vi "vPage_9205x1_CHx4.vi"() -> ()   [LabVIEW 2022 SP3]
uses:
  <vilib>/Utility/sysdir.llb/System Directory Type.ctl
  <vilib>/express/express analysis/Spectral/Block/exnSpectralBlock spectral measurements peak poly.vi
  <vilib>/express/express analysis/Spectral/Block/exnSpectralBlock spectral measurements peak DDT.vi
  <vilib>/express/express analysis/Spectral/XNode/ExpressSpectralMeasurementsBlockNode.xnode
panel:
  in  "Show_FFT":bool
  in  "Show":bool
  in  "¸ê®Æ§¨\nµù°O>":string
  in  "Filter(Hz)\nLow-Cut":dbl=10.0
  out "DAQ Stoped":bool
  in  "SW \n(C1)":bool[](array[boolean])=[TRUE, TRUE, TRUE, TRUE, TRUE, TRUE, TRUE, TRUE]
  in  "Sample \nto Read":i32=6400
  in  "Sample\nRate":dbl=6400.0
  in  "Enable Saving":bool
  in  "Stop":bool
  out "C1-Save":bool
  out "C1-Trigger":bool
  out "C1":i32
  out "C1-All":dynamicdata(graph)
  out "C1-0":dynamicdata(graph)
  out "C1-2":dynamicdata(graph)
  out "C1-1":dynamicdata(graph)
  out "C1-3":dynamicdata(graph)
  # "使用前請先確認 \nDAQ 擷取卡設定"
  # "本頁畫面顯示為 觸發後訊號"
  # "FFT Filter by useing High-pass with Lower Cut-Off (Hz)"
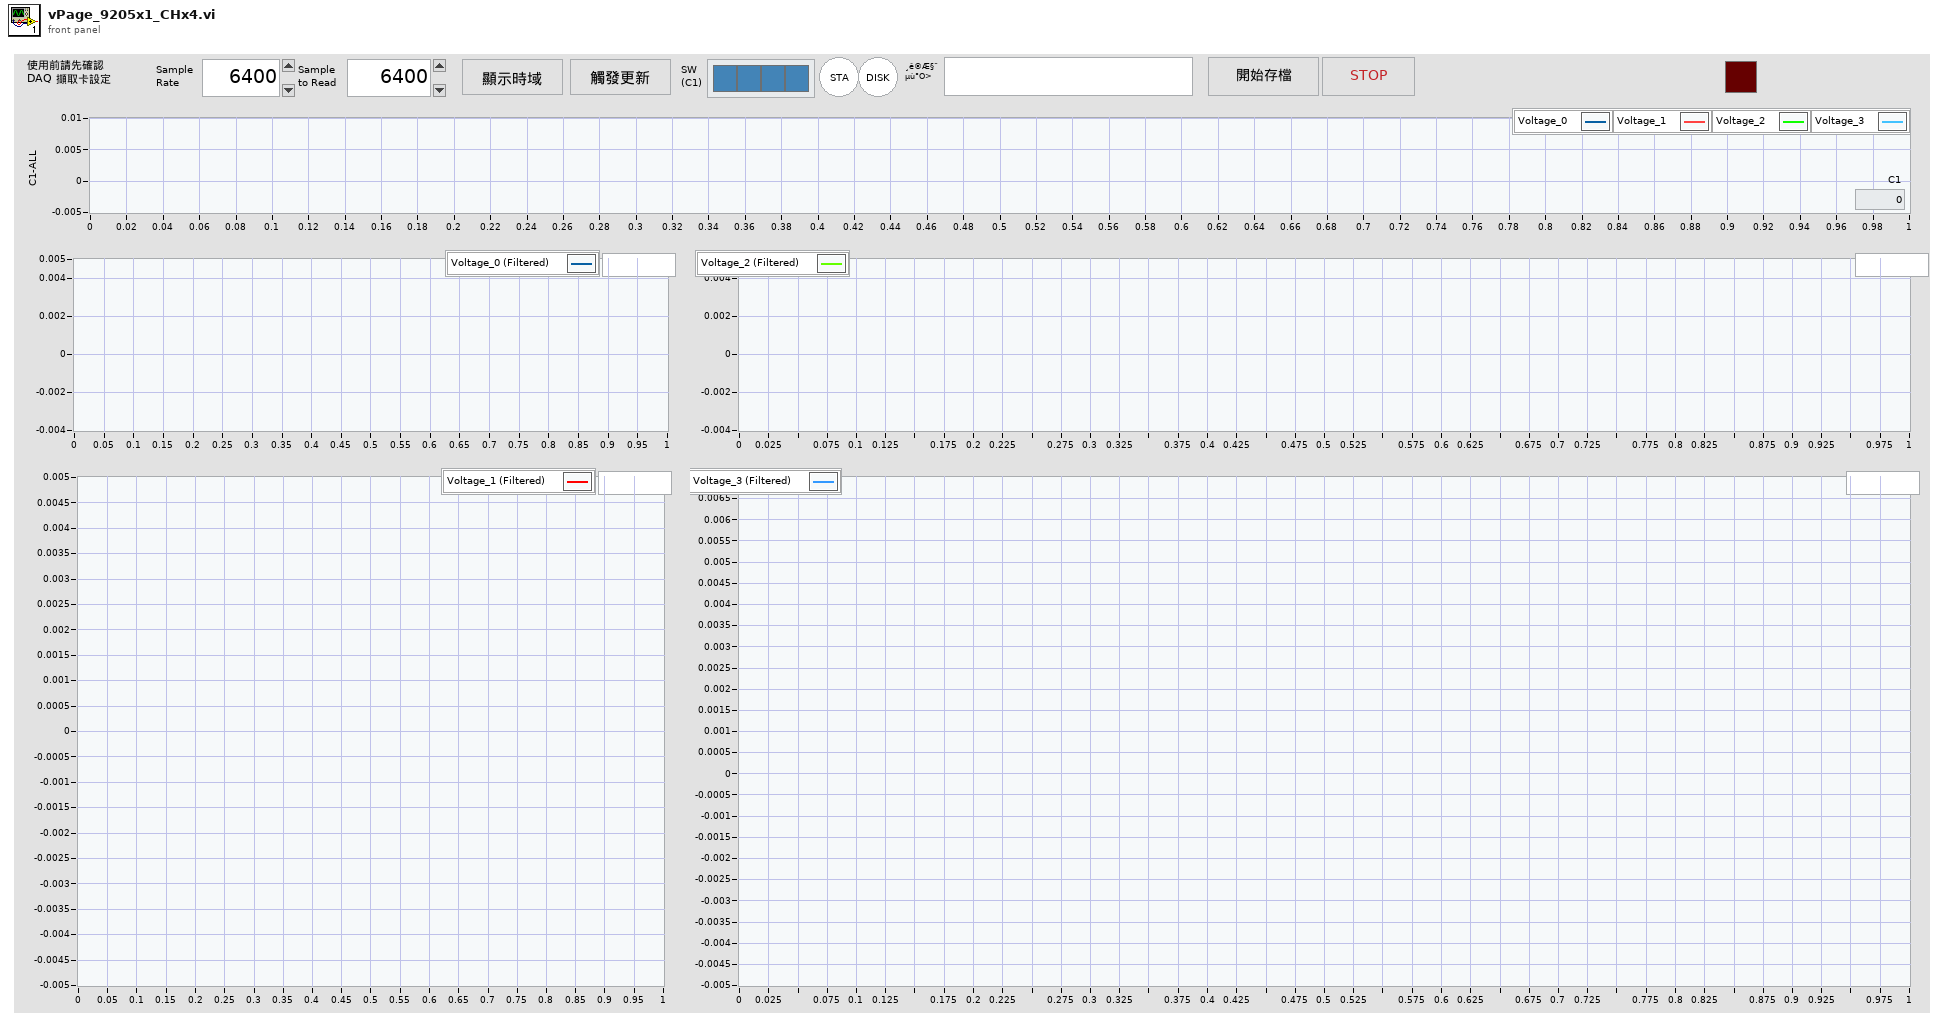
[diagram p1: front panel]
types:
  T1 = enum8{"Enabled", "Disabled", "Disabled and Grayed Out"}
  T2 = typedef "System Directory Type.ctl" = i32
  T3 = cluster{"task out":refnum<k21>, "data":dynamicdata}
  T4 = cluster{"averaging mode":u16, "weighting mode":u16, "number of averages":u32}
  T5 = cluster{"dB On (F)":bool, "unwrap phase (F)":bool, "convert to degree (F)":bool}
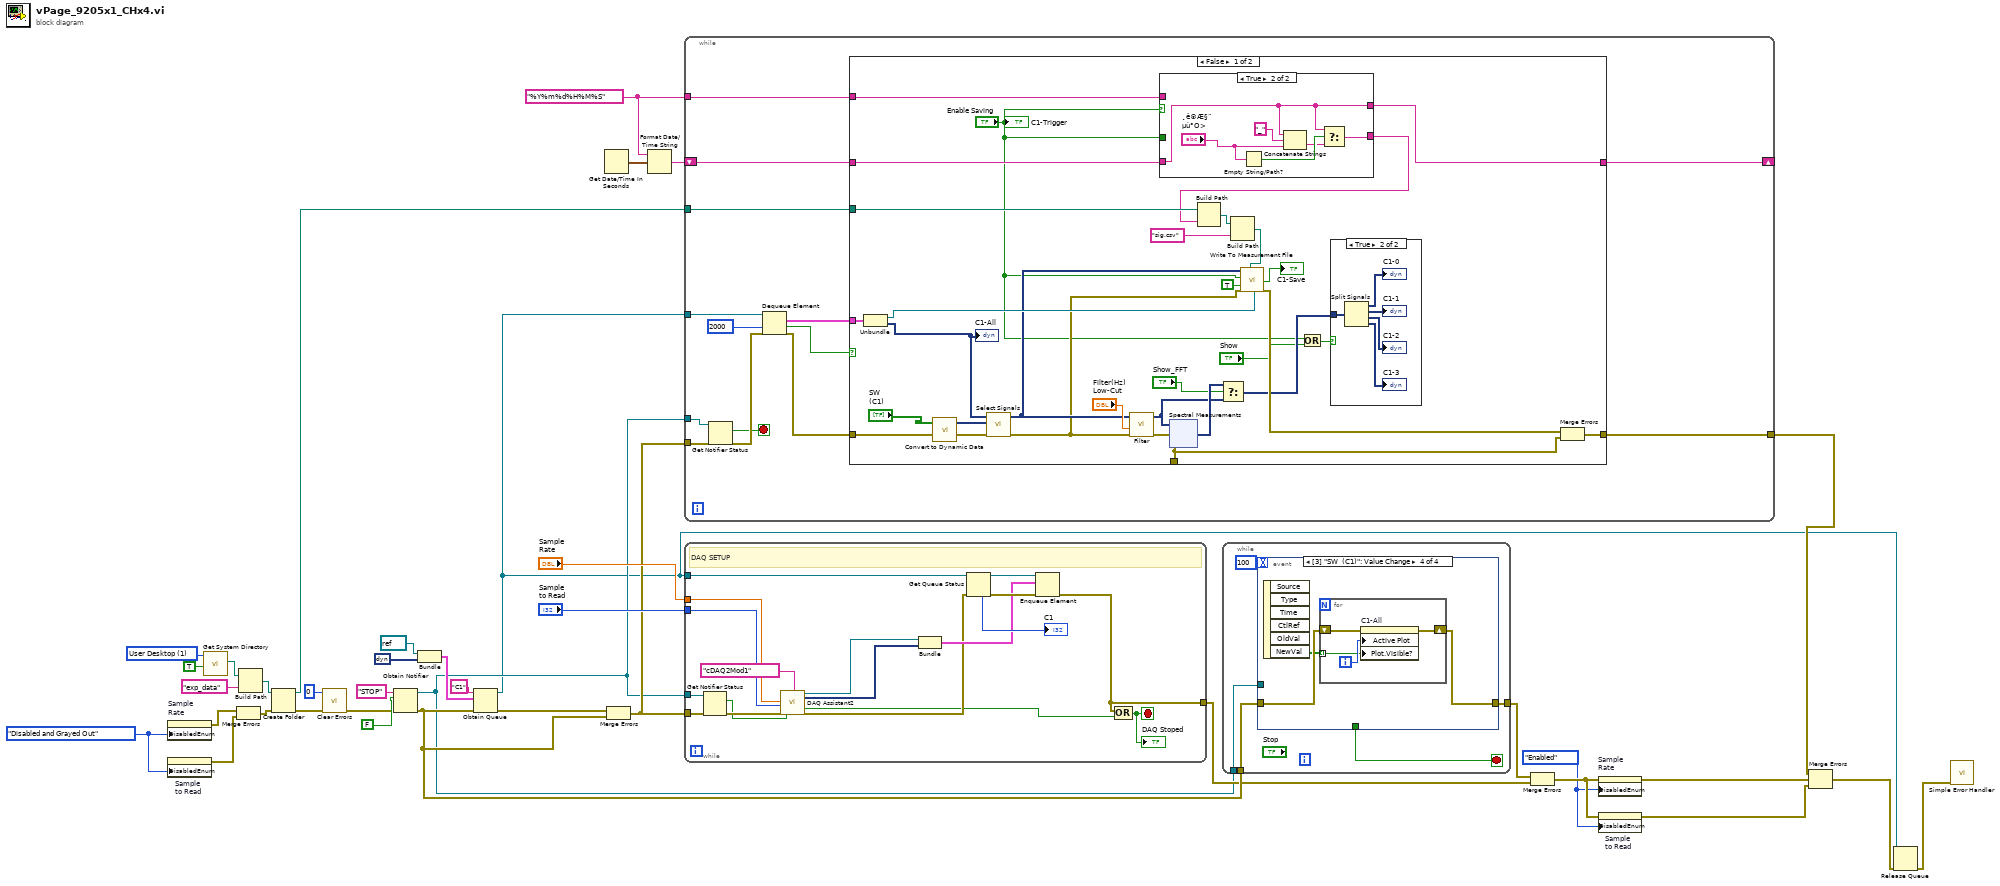
[diagram p0: block diagram]
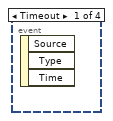
[diagram p2: hidden frame]
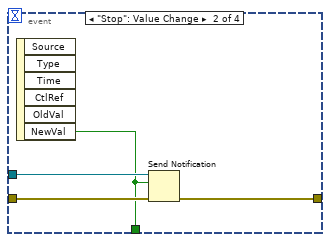
[diagram p3: hidden frame]
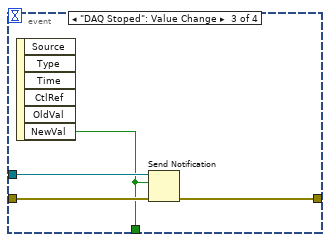
[diagram p4: hidden frame]
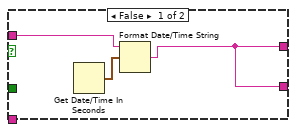
[diagram p6: hidden frame]
diagram:
  w7 = T1."Enabled" ("Disabled")
  w12 = T1."Disabled and Grayed Out" ("Disabled")
  w13 = "%Y%m%d%H%M%S" ("time format string (%c)")
  w23 = T2 1 items=["User Home"=0, "User Desktop"=1, "User Documents"=2, "User Application Data"=3, "User Preferences"=4, "User Temporary"=5, "Public Documents"=6, "Public Application Data"=7, "Public Preferences"=8, "Public Cache"=13, "System Core Libraries"=9, "System Installed Libraries"=10, "Application Files"=11, "Boot Volume Root"=12] ("system directory type")
  n1 = property on="Sample\nRate" class="DigNum (strict)"("DisabledEnum"=w12) -> (error out=w11:errorcluster)  [unwired: 2 in, 1 out]
  n2 = property on="Sample \nto Read" class="DigNum (strict)"("DisabledEnum"=w12) -> (error out=w9:errorcluster)  [unwired: 2 in, 1 out]
  n3 = call <vilib>:"Get System Directory.vi"("create directory if not found? (F)"=TRUE, "system directory type"=w23) -> ("system directory"=w25:path)  [unwired: 9 in]
  n4 = Merge Errors(w11, w9) -> (w10:errorcluster)
  n5 = Build Path(base path=w25, name or relative path="exp_data") -> (appended path=w19:path)
  n6 = Create Folder(path (use dialog)=w19, error in=w10) -> (created path=w18:path, error out=w21:errorcluster)  [unwired: 1 in, 1 out]
  n7 = call <vilib>:"Clear Errors.vi"("error in (no error)"=w21, "specific error code to clear (0: all)"=0) -> ("error out"=w20:errorcluster)  [unwired: 4 in, 1 out]
  n8 = Obtain Notifier(name (unnamed)="STOP", notification data type=FALSE, error in (no error)=w20) -> (notifier out=w14:refnum<notifier>, error out=w17:errorcluster)  [unwired: 1 in, 1 out]
  n9 = Bundle("task out"=refnum<k21> refnum, "data"=dynamicdata []) -> (w30:T3)  [unwired: 1 in]
  n10 = Obtain Queue(name (unnamed)="C1", element data type=w30, error in (no error)=w17) -> (queue out=w1:refnum<queue>, error out=w38:errorcluster)  [unwired: 2 in, 1 out]
  n11 = Get Date/Time In Seconds() -> (seconds since 1Jan1904=w28:timestamp)
  n12 = Merge Errors(w38, w17) -> (w29:errorcluster)
  n13 = Format Date/Time String(time format string (%c)=w13, seconds (now)=w28) -> (date/time string=w27:string)  [unwired: 1 in]
  n14 = while {
    tunnel: w29 -> [w52]
    tunnel: w14 -> [w50]
    tunnel: w1 -> [w49]
    shift-right: [w39] -> _
    shift-left: w27 -> [w43]
    tunnel: w18 -> [w44]
    tunnel: [w40] -> w2
    tunnel: w13 -> [w42]
    stop <- w47 stop-if-true
    n15 = Get Notifier Status(notifier=w50, error in (no error)=w52) -> (current notification=w47:bool, error out=w51:errorcluster)  [unwired: 3 out]
    n16 = Dequeue Element(queue=w49, timeout in ms (-1)=2000, error in (no error)=w51) -> (element=w45:T3, timed out?=w46:bool, error out=w41:errorcluster)  [unwired: 1 out]
    n17 = case shown="False" w46 {
      tunnel: w45 -> [w80 _]
      tunnel: w41 -> [w79 w107]
      tunnel: [w68 _] -> _
      tunnel: w43 -> [w75 w108]
      tunnel: [w74 w108] -> w39
      tunnel: w44 -> [w73 _]
      tunnel: [w67 w107] -> w40
      tunnel: w42 -> [w60 _]
      frame False {
        n18 = Unbundle(w80) -> ("task out"=w78:refnum<k21>, "data"=w55:dynamicdata)
        "C1-All" <- w55
        n19 = call "Convert to Dynamic Data"("Array"="SW \n(C1)") -> ("Dynamic Data Type"=w64:dynamicdata)  [unwired: 3 in]
        n20 = call "Select Signals"("error in (no error)"=w79, "Selector Input"=w64, "Signals"=w55) -> ("error out"=w76:errorcluster, "Signal Out"=w77:dynamicdata)  [unwired: 7 in]
        n21 = call "Filter"("error in (no error)"=w76, "Lower Cut-Off"="Filter(Hz)\nLow-Cut", "Signal"=w77) -> ("error out"=w82:errorcluster, "Filtered Signal"=w65:dynamicdata)  [unwired: 7 in]
        n22 = case shown="True" "Enable Saving" {
          tunnel: [w88 w92] -> w74
          tunnel: "Enable Saving" -> [_ _]
          tunnel: w75 -> [_ w92]
          tunnel: [w88 w94] -> w61
          tunnel: w60 -> [w89 _]
          frame False {
            n23 = Get Date/Time In Seconds() -> (seconds since 1Jan1904=w90:timestamp)
            n24 = Format Date/Time String(time format string (%c)=w89, seconds (now)=w90) -> (date/time string=w88:string)  [unwired: 1 in]
          }
          frame True {
            n25 = Empty String/Path?(string/path="¸ê®Æ§¨\nµù°O>") -> (empty?=w96:bool)
            n26 = Concatenate Strings(w92, "_" ("string"), "¸ê®Æ§¨\nµù°O>") -> (w95:string)
            n27 = Select(t=w92, s=w96, f=w95) -> (s? t:f=w94:string)
          }
        }
        n28 = xnode ("Spectral Measurements")("Signals"=w65, "error in (no error)"=w82) -> ("FFT - (Peak)"=w66:dynamicdata, "error out"=w68:errorcluster)  [unwired: 1 out]
        n29 = Build Path(base path=w73, name or relative path=w61) -> (appended path=w72:path)
        n30 = Select(t=w66, s="Show_FFT", f=w65) -> (s? t:f=w63:dynamicdata)
        n31 = Build Path(base path=w72, name or relative path="sig.csv") -> (appended path=w70:path)
        n32 = call "Write To Measurement File"("Signals"=w77, "Enable"="Enable Saving", "new_file"=TRUE, "error in (no error)"=w76, "Filename"=w70, "DAQmx Task"=w78) -> ("Saving Data"=→"C1-Save":bool, "error out"=w69:errorcluster)  [unwired: 11 in, 1 out]
        n33 = Or(x="Enable Saving", y="Show") -> (x .or. y?=w59:bool)
        n34 = case shown="True" w59 {
          tunnel: w63 -> [_ w84]
          frame False {
          }
          frame True {
            n35 = Split Signals(w84) -> (→"C1-0":dynamicdata, →"C1-1":dynamicdata, →"C1-2":dynamicdata, →"C1-3":dynamicdata)  [unwired: 4 in]
          }
        }
        n36 = Merge Errors(w69, w68) -> (w67:errorcluster)
        "C1-Trigger" <- "Enable Saving"
      }
      frame True {
      }
    }
  }
  n37 = while {
    tunnel: [w125] -> w15
    tunnel: w1 -> [w122]
    tunnel: w29 -> [w121]
    tunnel: w14 -> [w120]
    tunnel: "Sample \nto Read" -> [w114]
    tunnel: "Sample\nRate" -> [w115]
    stop <- w123 stop-if-true
    # "DAQ SETUP"
    n38 = Get Notifier Status(notifier=w120, error in (no error)=w121) -> (current notification=w113:bool, error out=w117:errorcluster)  [unwired: 3 out]
    n39 = call "DAQ Assistant2"("rate"=w115, "number of samples"=w114, "error in"=w117, "stop (F)"=w113, "device name"=tag "cDAQ2Mod1") -> ("task out"=w111:refnum<k21>, "data"=w110:dynamicdata, "stopped"=w112:bool, "error out"=w116:errorcluster)  [unwired: 11 in]
    n40 = Bundle("task out"=w111, "data"=w110) -> (w118:T3)  [unwired: 1 in]
    n41 = Get Queue Status(queue=w122, error in (no error)=w116) -> (queue out=w119:refnum<queue>, error out=w126:errorcluster, # elements in queue=→"C1":i32)  [unwired: 1 in, 5 out]
    n42 = Enqueue Element(queue=w119, element=w118, error in (no error)=w126) -> (error out=w125:errorcluster)  [unwired: 1 in, 2 out]
    n43 = Compound Arithmetic op=OR(w125, w112) -> (w123:bool)
    "DAQ Stoped" <- w123
  }
  n44 = while {
    tunnel: w17 -> [w131]
    tunnel: [w130] -> w16
    tunnel: w14 -> [w129]
    stop <- w128 stop-if-true
    n45 = event shown="[3] \"SW  (C1)\": Value Change" {
      selector: _ -> [_ _ _ _]
      dyn-events: _ -> [_ _ _ _]
      timeout: 100 -> [_ _ _ _]
      tunnel: w131 -> [_ w135 w139 w142]
      tunnel: [_ w134 w138 w141] -> w130
      tunnel: w129 -> [_ w133 w137 _]
      tunnel: [_ w132 w136 _] -> w128
      event Timeout {
        n46 = event-data() -> ()  [unwired: 1 in, 3 out]
      }
      event "Stop": Value Change {
        n47 = event-data() -> ("NewVal"=w132:bool)  [unwired: 1 in, 5 out]
        n48 = Send Notification(notification=w132, notifier=w133, error in (no error)=w135) -> (error out=w134:errorcluster)  [unwired: 1 out]
      }
      event "DAQ Stoped": Value Change {
        n49 = event-data() -> ("NewVal"=w136:bool)  [unwired: 1 in, 5 out]
        n50 = Send Notification(notification=w136, notifier=w137, error in (no error)=w139) -> (error out=w138:errorcluster)  [unwired: 1 out]
      }
      event "SW \n(C1)": Value Change {
        n51 = event-data() -> ("NewVal"=w140:bool[])  [unwired: 1 in, 5 out]
        n52 = for {
          shift-right: [w143] -> w141
          shift-left: w142 -> [w145]
          tunnel: w140 -> [w144] mode=indexing
          i -> [w146]
          n53 = property on="C1-All" class="WFGraph (strict)"(error in=w145, "Active Plot"=w146, "Plot.Visible?"=w144) -> (error out=w143:errorcluster)  [unwired: 1 in, 1 out]
        }
      }
    }
  }
  n54 = Merge Errors(w16, w15) -> (w8:errorcluster)
  n55 = property on="Sample\nRate" class="DigNum (strict)"(error in=w8, "DisabledEnum"=w7) -> (error out=w6:errorcluster)  [unwired: 1 in, 1 out]
  n56 = property on="Sample \nto Read" class="DigNum (strict)"(error in=w8, "DisabledEnum"=w7) -> (error out=w5:errorcluster)  [unwired: 1 in, 1 out]
  n57 = Merge Errors(w2, w6, w5) -> (w3:errorcluster)
  n58 = Release Queue(queue=w1, error in (no error)=w3) -> (error out=w4:errorcluster)  [unwired: 1 in, 2 out]
  n59 = call <vilib>:"Simple Error Handler.vi"("error in (no error)"=w4) -> ()  [unwired: 4 in, 5 out]
